vi "lab3_exp1.vi"() -> ()   [LabVIEW 2015]
uses:
  <vilib>/measure/NI_MABase.lvlib
panel:
  out "Filtered Signal Graph":dynamicdata(graph)=[{"t0"=timestamp(0 s since 1904-01-01), "dt"=0.001, "Y"=array[1000 elements], "attributes"=variant("NI_ChannelName"=variant(string "Filtered"))}]
  out "Sine  + Random Signal Graph":waveform(dbl)(graph)={"t0"=timestamp(0 s since 1904-01-01), "dt"=0.001, "Y"=array[2000 elements]}
  in  "sampling info":cluster{"Fs":dbl, "#s":dbl}={"Fs"=1000.0, "#s"=2000.0} {"Fs" format="%.2p"}
  out "Sine Wave Graph":waveform(dbl)(graph)={"t0"=timestamp(0 s since 1904-01-01), "dt"=0.001, "Y"=array[2000 elements]}
  in  "amplitude":dbl=1.0 format="%0.2p"
  in  "frequency":dbl=10.0 format="%0.2p"
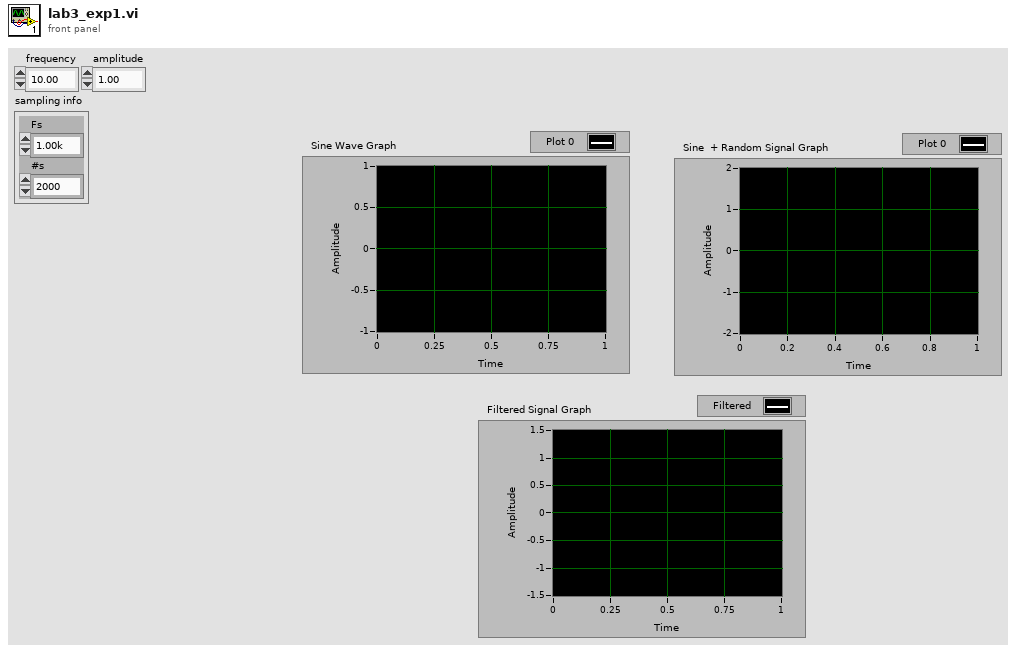
[diagram p1: front panel]
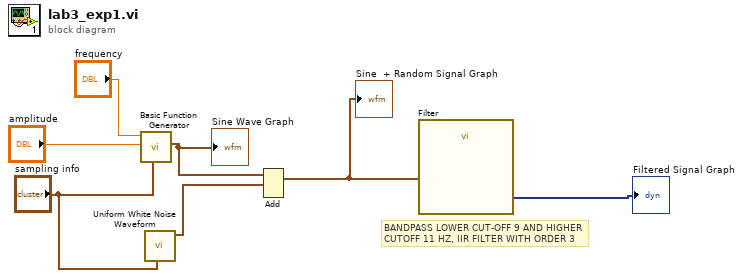
[diagram p0: block diagram]
diagram:
  # "BANDPASS LOWER CUT-OFF 9 AND HIGHER CUTOFF 11 HZ, IIR FILTER WITH ORDER 3"
  n1 = call <vilib>:"Basic Function Generator.vi"("sampling info"="sampling info", "amplitude"="amplitude", "frequency"="frequency") -> ("signal out"=w4:waveform(dbl))  [unwired: 6 in, 2 out]
  "Sine Wave Graph" <- w4
  n2 = call <vilib>:"Uniform White Noise Waveform.vi"("sampling info"="sampling info") -> ("signal out"=w3:waveform(dbl))  [unwired: 9 in, 1 out]
  n3 = Add(1:w3, 2:w4) -> (0:w1:waveform(dbl))  [unwired: 1 in, 1 out]
  "Sine  + Random Signal Graph" <- w1
  n4 = call "Filter"("Signal"=w1) -> ("Filtered Signal"=→"Filtered Signal Graph":dynamicdata)  [unwired: 9 in, 1 out]
